vi "pre_scan.vi"(6 "scan_values":dbl[](array[numeric]), 7 "wait (ms)":i32=1000, 8 "error in (no error)":errorcluster) -> (0 "error out":errorcluster)   [LabVIEW 2017, in "sirah.lvlib"]
uses:
  sirah.lvlib
panel:
  # "Set first value and wait 1 s."
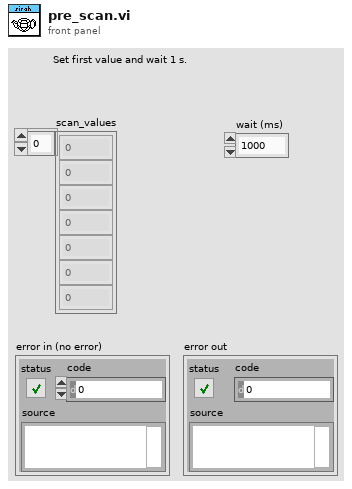
[diagram p1: front panel]
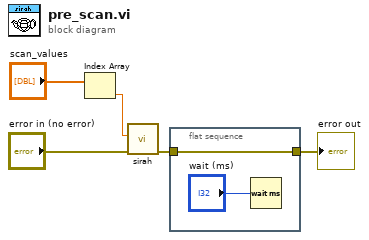
[diagram p0: block diagram]
diagram:
  n1 = Index Array(array="scan_values") -> (element=w1:dbl)  [unwired: 1 in]
  n2 = call "sirah.vi"("error in (no error)"="error in (no error)", "wavelength (nm)"=w1) -> ("error out"=w3:errorcluster)  [unwired: 7 in, 2 out]
  n3 = flat-sequence {
    tunnel: [w7] -> w4
    tunnel: w3 -> [w7]
    frame #0 {
      n4 = Wait (ms)(milliseconds to wait="wait (ms)") -> ()  [unwired: 1 out]
    }
  }
  "error out" <- w4
